vi "voltageSet.vi"(4 "error in (no error)":errorcluster, 5 "SEQ in":u32, 6 "Voltage":sgl, 7 "connection ID":refnum<k5>) -> (0 "error out":errorcluster, 1 "SEQ out":u32, 2 "OK？":bool, 3 "connection ID out":refnum<k5>)   [LabVIEW 2016]
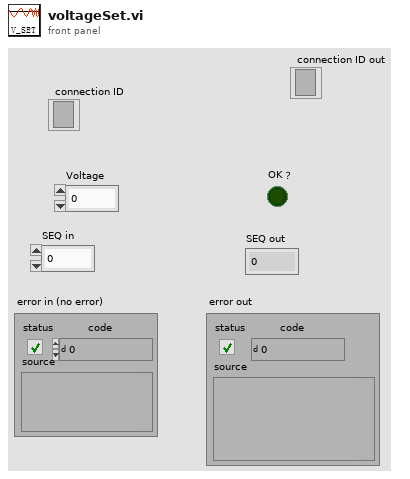
[diagram p1: front panel]
types:
  T1 = enum8{"SET_FREQ", "SET_VOLT", "SET_CHANNEL_VOLT", "SET_PHASE", "START_HEAT", "STOP_HEAT", "CHANNEL_CTRL_SINGLE", "CHANNEL_CTRL_ALL", "READ_VOLT_SET", "READ_VOLT_SET_RSP", "READ_CURRENT_VOLT", "READ_CURRENT_VOLT_RSP", "READ_PHASE", "READ_PHASE_RSP", "READ_HEATTIME_LEFT", "READ_HEATTIME_LEFT_RSP", "EXEC_RSP"}
  T2 = enum8{"SET_FREQ", "SET_VOLT", "SET_CHENNEL_VOLT", "SET_PHASE", "START_HEAT", "STOP_HEAT", "CHANNEL_CTRL_SINGLE", "CHANNEL_CTRL_ALL", "READ_VOLT_SET", "READ_VOLT_SET_RSP", "READ_CURRENT_VOLT", "READ_CURRENT_VOLT_RSP", "READ_PHASE", "READ_PHASE_RSP", "READ_HEATTIME_LEFT", "READ_HEATTIME_LEFT_RSP", "EXEC_RSP"}
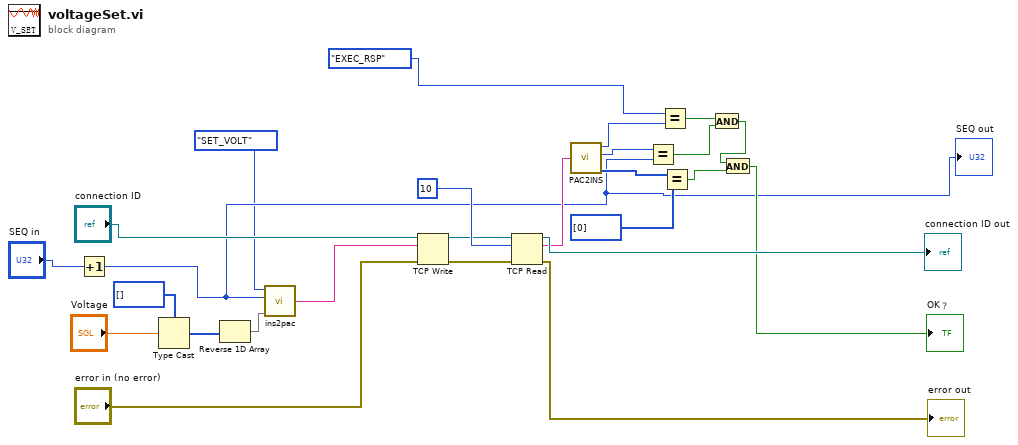
[diagram p0: block diagram]
diagram:
  n1 = Increment(x="SEQ in") -> (x+1=w6:u32)
  "SEQ out" <- w6
  n2 = Type Cast(type=u8[] [], x="Voltage") -> (*(type *) &x=w4:u8[])
  n3 = Reverse 1D Array(array=w4) -> (reversed array=w3:u8[])
  n4 = call "ins2pac.vi"("BODY"=w3, "SEQUENCE"=w6, "TYPE"=T1."SET_VOLT") -> ("PACKET"=w23:string)  [unwired: 1 in]
  n5 = TCP Write(connection ID="connection ID", data in=w23, error in (no error)="error in (no error)") -> (connection ID out=w20:refnum<k5>, error out=w19:errorcluster)  [unwired: 1 in, 1 out]
  n6 = TCP Read(connection ID=w20, bytes to read=10, error in (no error)=w19) -> (connection ID out=→"connection ID out":refnum<k5>, data out=w16:string, error out=→"error out":errorcluster)  [unwired: 2 in]
  n7 = call "PAC2INS.vi"("PACKET"=w16) -> ("TYPE"=w15:T2, "SEQUENCE"=w14:u32, "BODY"=w13:u8[])  [unwired: 1 out]
  n8 = Equal?(x=w14, y=w6) -> (x = y?=w10:bool)
  n9 = Equal?(x=T1."EXEC_RSP" ("TYPE"), y=w15) -> (x = y?=w11:bool)
  n10 = Equal?(x=w13, y=u8[] [0]) -> (x = y?=w8:bool)
  n11 = And(x=w11, y=w10) -> (x .and. y?=w9:bool)
  n12 = And(x=w9, y=w8) -> (x .and. y?=→"OK？":bool)
